vi "Find Range Check Result by Name.vi"(8 "error in":errorcluster, 10 "Device Name":string, 11 "Range Check Results in":T1(array[cluster])=[{"name"="D:OUTTMP", "value"=17.051272696256788, "range state"=0}]) -> (0 "error out":errorcluster, 2 "Found?":bool, 3 "Range Check Result out":T2)   [LabVIEW 2013, in "ACNET Monitor.lvlib"]
uses:
  ACNET Monitor.lvlib
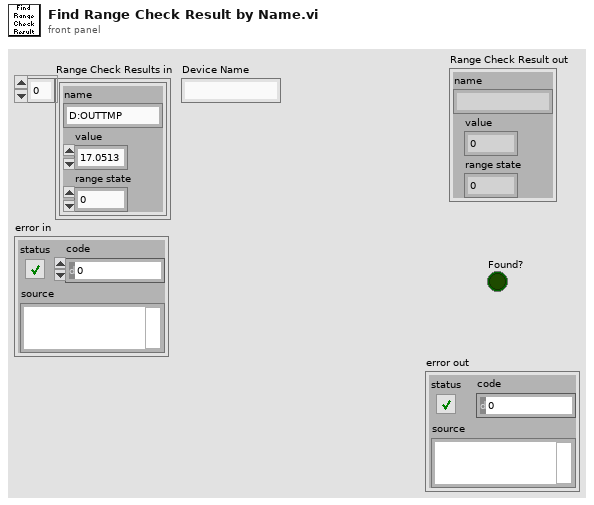
[diagram p1: front panel]
types:
  T1 = cluster{"name":string, "value":dbl, "range state":i8}[]
  T2 = cluster{"name":string, "value":dbl, "range state":i8}
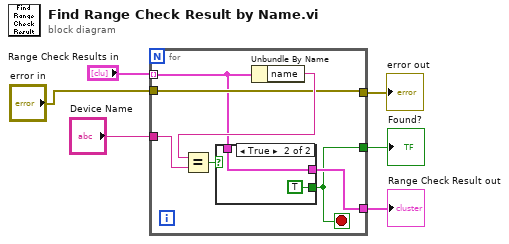
[diagram p0: block diagram]
diagram:
  n1 = for {
    tunnel: "Range Check Results in" -> [w7] mode=indexing
    tunnel: "error in" -> [w8]
    tunnel: "Device Name" -> [w12]
    tunnel: [w8] -> w4
    tunnel: [w10] -> w5
    tunnel: [w9] -> w6
    stop <- w9 stop-if-true
    n2 = Unbundle By Name(w7) -> ("name"=w13:string)
    n3 = Equal?(x=w13, y=w12) -> (x = y?=w11:bool)
    n4 = case shown="True" w11 {
      tunnel: [_ TRUE] -> w9
      tunnel: w7 -> [_ w14]
      tunnel: [_ w14] -> w10
      frame False {
      }
      frame True {
      }
    }
  }
  "error out" <- w4
  "Range Check Result out" <- w5
  "Found?" <- w6
